vi "SecondaryRobotFunctions.vi"(5 "Drive Joystick Values":dbl[](array[numeric]), 6 "Robot State":T1, 7 "Automatic State Control Mode (F)":bool, 8 "Secondary Joystick Values":dbl[](array[numeric]), 9 "ADIS Gyro Values":T9 {"IMU Data Out"."X Accel (g)" format="%#_3g"; "IMU Data Out"."Y Accel (g)" format="%#_3g"; "IMU Data Out"."Z Accel (g)" format="%#_3g"}, 10 "Drive Joystick Buttons":bool[](array[boolean]), 11 "Secondary Joystick Buttons":bool[](array[boolean])) -> ()   [LabVIEW 2019]
uses:
  Controls/ADIS Gyro Values.ctl
  Controls/Robot State.ctl
  Controls/Robot Pivot Motion Commands.ctl
  Controls/Pivot Motor Commands.ctl
  Controls/Robot Drive Mode.ctl
  Controls/Enable Actions.ctl
  Controls/Lift System Actions.ctl
  Controls/Spinner Actions.ctl
  Controls/Ball System Actions.ctl
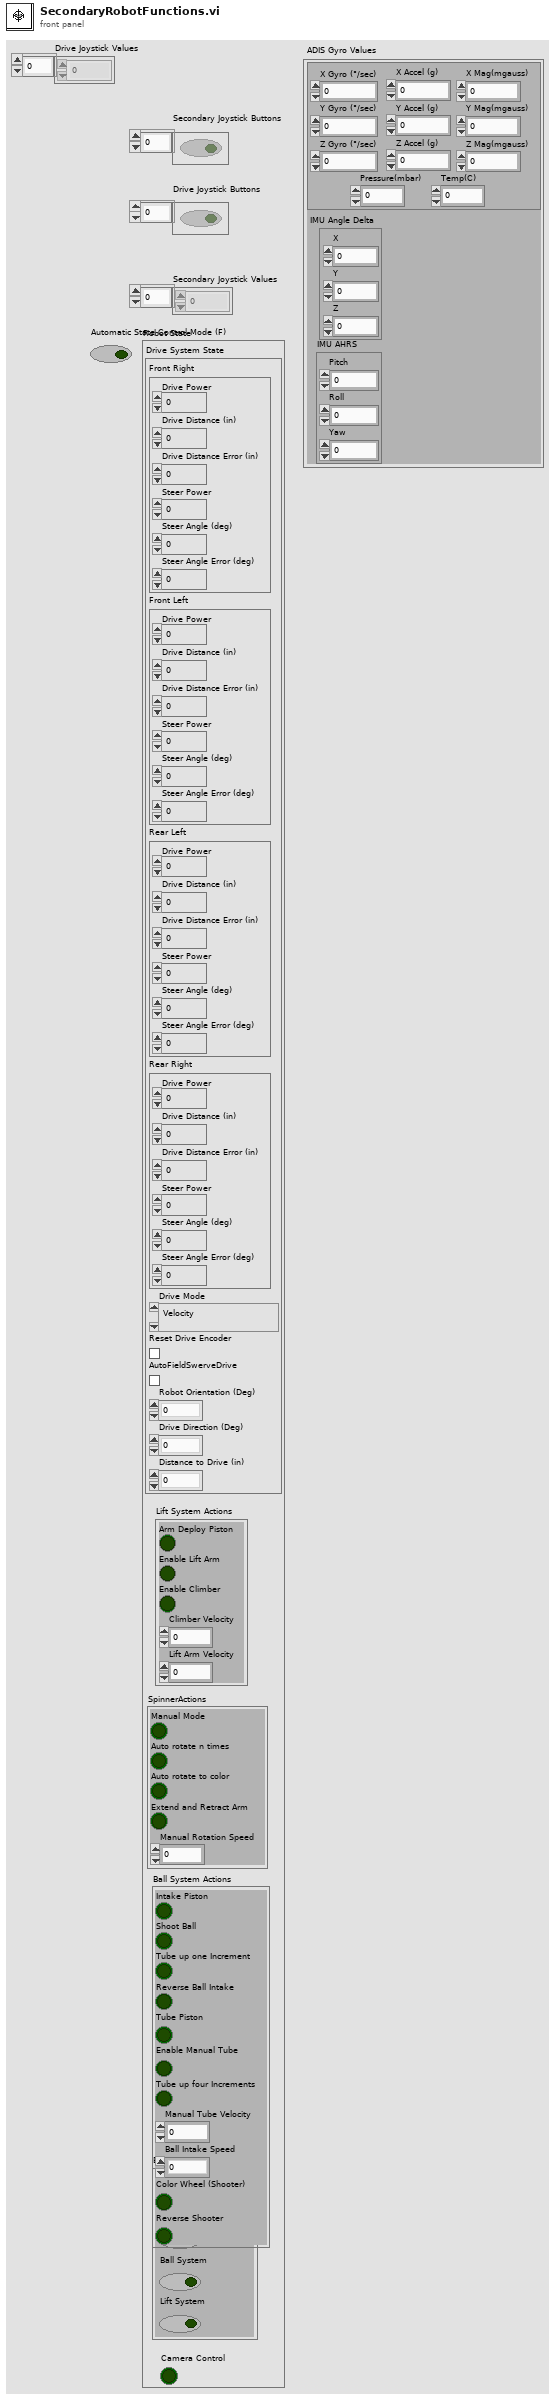
[diagram p1: front panel]
types:
  T1 = typedef "Robot State.ctl" = cluster{"Drive System State":T2, "Enable Actions":T5, "Lift System Actions":T6, "SpinnerActions":T7, "Ball System Actions":T8, "Camera Control":bool}
  T2 = typedef "Robot Pivot Motion Commands.ctl" = cluster{"Front Right":T3, "Front Left":T3, "Rear Left":T3, "Rear Right":T3, "Drive Mode":T4, "Reset Drive Encoder":bool, "AutoFieldSwerveDrive":bool, "Robot Orientation (Deg)":dbl, "Drive Direction (Deg)":dbl, "Distance to Drive (in)":dbl}
  T3 = typedef "Pivot Motor Commands.ctl" = cluster{"Drive Power":dbl, "Drive Distance (in)":dbl, "Drive Distance Error (in)":dbl, "Steer Power":dbl, "Steer Angle (deg)":dbl, "Steer Angle Error (deg)":dbl}
  T4 = typedef "Robot Drive Mode.ctl" = enum16{"Velocity", "Distance"}
  T5 = typedef "Enable Actions.ctl" = cluster{"Manual Swerve Drive":bool, "Color System":bool, "Ball System":bool, "Lift System":bool}
  T6 = typedef "Lift System Actions.ctl" = cluster{"Arm Deploy Piston":bool, "Enable Lift Arm":bool, "Enable Climber":bool, "Climber Velocity":dbl, "Lift Arm Velocity":dbl}
  T7 = typedef "Spinner Actions.ctl" = cluster{"Manual Mode ":bool, "Auto rotate n times":bool, "Auto rotate to color\t":bool, "Extend and Retract Arm\t":bool, "Manual Rotation Speed":dbl}
  T8 = typedef "Ball System Actions.ctl" = cluster{"Intake Piston ":bool, "Shoot Ball":bool, "Tube up one Increment\t":bool, "Reverse Ball Intake":bool, "Tube Piston":bool, "Enable Manual Tube":bool, "Tube up four Increments":bool, "Manual Tube Velocity":dbl, "Ball Intake Speed":dbl, "Color Wheel (Shooter)":bool, "Reverse Shooter":bool}
  T9 = typedef "ADIS Gyro Values.ctl" = cluster{"IMU Data Out":cluster{"X Gyro (°/sec)":dbl, "Y Gyro (°/sec)":dbl, "Z Gyro (°/sec)":dbl, "X Accel (g)":dbl, "Y Accel (g)":dbl, "Z Accel (g)":dbl, "X Mag(mgauss)":dbl, "Y Mag(mgauss)":dbl, "Z Mag(mgauss)":dbl, "Pressure(mbar)":dbl, "Temp(C)":dbl}, "IMU Angle Delta":cluster{"X":dbl, "Y":dbl, "Z":dbl}, "IMU AHRS":cluster{"Pitch":dbl, "Roll":dbl, "Yaw":dbl}}
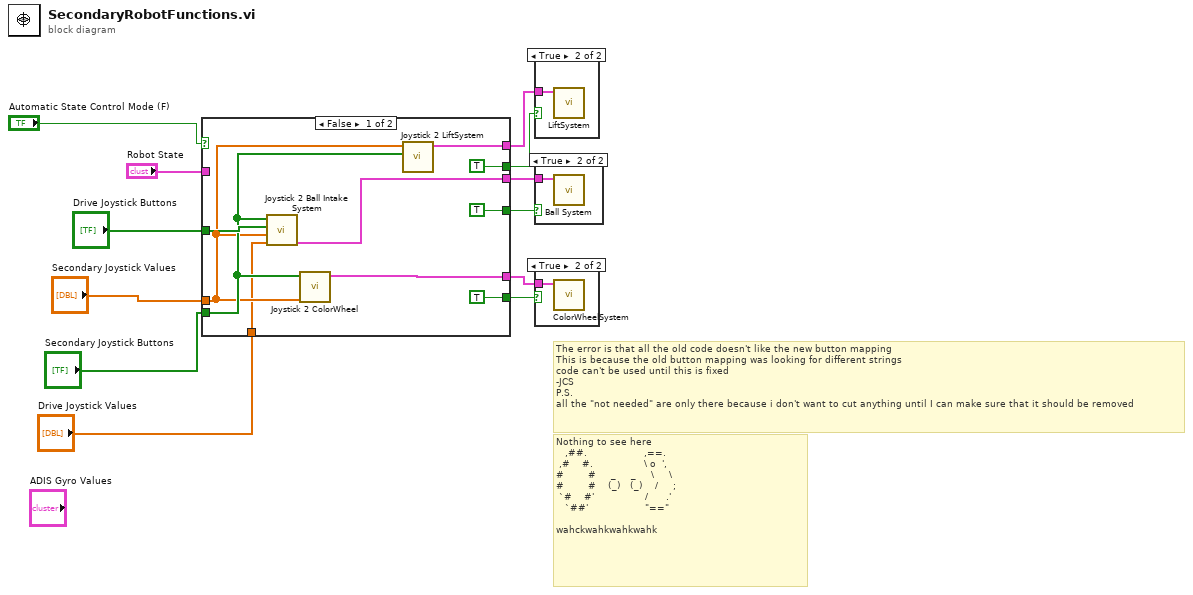
[diagram p0: block diagram]
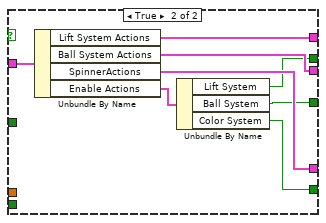
[diagram p5: hidden frame]
diagram:
  # "Nothing to see here\n   ,##.                   ,==.\n ,#    #.                 \\ o  ',\n#        #     _     _     \\     \\\n#        #    (_)   (_)    /     ; \n `#    #'                 /      .'  \n   `##'                   \"==\"\n\nwahckwahkwahkwahk"
  # "The error is that all the old code doesn't like the new button mapping\nThis is because the old button mapping was looking for different strings\ncode can't be used until this is fixed\n-JCS\nP.S. \nall the \"not needed\" are only there because i don't want to cut anything until I can make sure that it should be removed"
  n1 = case shown="False" "Automatic State Control Mode (F)" {
    tunnel: "Secondary Joystick Buttons" -> [w15 _]
    tunnel: "Secondary Joystick Values" -> [w14 _]
    tunnel: [w22 w29] -> w10
    tunnel: "Robot State" -> [_ w30]
    tunnel: [TRUE w25] -> w7
    tunnel: [TRUE ("Ball Intake") w24] -> w6
    tunnel: [TRUE w23] -> w5
    tunnel: [w19 w27] -> w4
    tunnel: [w18 w28] -> w3
    tunnel: "Drive Joystick Buttons" -> [w17 _]
    tunnel: "Drive Joystick Values" -> [w13 _]
    frame False {
      n2 = call "Joystick 2 Ball Intake System.vi"("Drive Joystick Values"=w13, "Secondary Joystick Values"=w14, "Drive Joystick Buttons"=w17, "Secondary Joystick Buttons"=w15) -> ("Ball System Actions"=w18:T8)  [unwired: 7 in]
      n3 = call "Joystick 2 ColorWheel.vi"("Secondary Joystick Values"=w14, "Secondary Joystick Buttons"=w15) -> ("SpinnerActions"=w19:T7)  [unwired: 9 in]
      n4 = call "Joystick 2 LiftSystem.vi"("Secondary Joystick Buttons"=w15, "JoystickAxes"=w14) -> ("Lift System Actions"=w22:T6)  [unwired: 9 in]
    }
    frame True {
      n5 = Unbundle By Name(w30) -> ("Lift System Actions"=w29:T6, "Ball System Actions"=w28:T8, "SpinnerActions"=w27:T7, "Enable Actions"=w26:T5)
      n6 = Unbundle By Name(w26) -> ("Lift System"=w25:bool, "Ball System"=w24:bool, "Color System"=w23:bool)
    }
  }
  n7 = case shown="True" w7 {
    tunnel: w10 -> [_ w31]
    frame False {
    }
    frame True {
      n8 = call "LiftSystem.vi"("Lift System Actions"=w31) -> ()  [unwired: 11 in]
    }
  }
  n9 = case shown="True" w6 {
    tunnel: w3 -> [_ w32]
    frame False {
    }
    frame True {
      n10 = call "Ball System.vi"("Ball System Actions"=w32) -> ()  [unwired: 10 in]
    }
  }
  n11 = case shown="True" w5 {
    tunnel: w4 -> [_ w33]
    frame False {
    }
    frame True {
      n12 = call "ColorWheelSystem.vi"("SpinnerActions"=w33) -> ()  [unwired: 11 in]
    }
  }
